vi "波形显示.vi"() -> ()   [LabVIEW 2019]
panel:
  out "波形图表":dbl(graph)
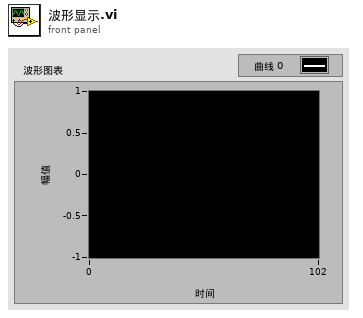
[diagram p1: front panel]
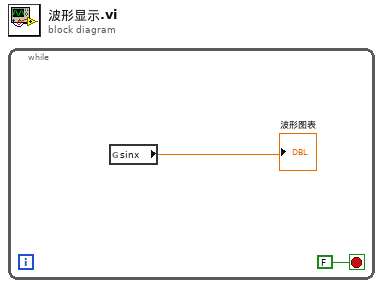
[diagram p0: block diagram]
diagram:
  n1 = while {
    stop <- FALSE stop-if-true
    n2 = global read "sinx.vi" "sinx"() -> (→"波形图表":dbl)
  }
